vi "GetValueForKey.vi"() -> ()   [LabVIEW 2018]
panel:
  out "error out":errorcluster
  in  "Key":string="everything"
  in  "Dictionary":cluster{"Key":string, "value":dbl}[](array[cluster])=[{"Key"="test", "value"=123.0}, {"Key"="test2", "value"=456.0}, {"Key"="everything", "value"=42.0}]
  out "value":dbl
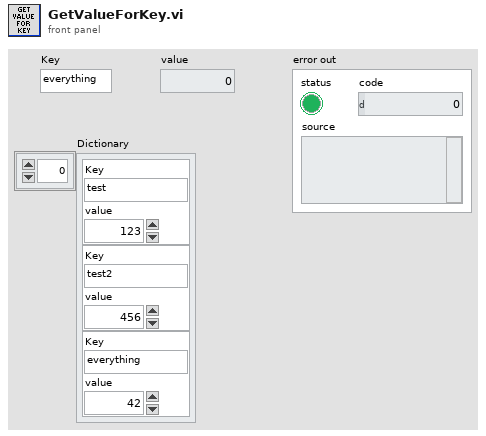
[diagram p1: front panel]
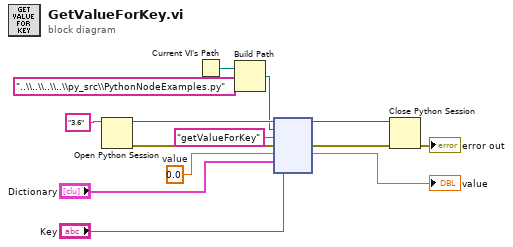
[diagram p0: block diagram]
diagram:
  w8 = 0.0  # value
  n1 = Open Python Session(python version="3.6" ("Python version")) -> (session out=w14:refnum<k35>, error out=w6:errorcluster)  [unwired: 2 in]
  n2 = Current VI's Path() -> (path=w5:path)
  n3 = Build Path(base path=w5, name or relative path="..\\..\\..\\..\\py_src\\PythonNodeExamples.py") -> (appended path=w3:path)
  n4 = node(w14, w3, "getValueForKey" ("function name"), w6, w8, "Dictionary", "Key") -> (w13:refnum<k35>, w2:errorcluster, →"value":dbl)  [unwired: 2 in, 2 out]
  n5 = Close Python Session(session in=w13, error in=w2) -> (11:→"error out":errorcluster)
